vi "Publish.vi"(8 "error in (no error)":errorcluster, 10 "PublishRequest":refnum<class "PublishRequest.lvclass">, 11 "Mediator in":refnum<class "Mediator.lvclass">) -> (0 "error out":errorcluster, 3 "Mediator out":refnum<class "Mediator.lvclass">)   [LabVIEW 2019, in "Mediator.lvlib" / "Mediator.lvclass"]
doc: "<License>\nCopyright © 2017 Composed Systems, LLC | All rights reserved\nwww.composed.io\n\nAuthor: Ethan Stern <ethan.stern@composed.io>\n\nThis software is provided \"AS IS\" WITHOUT WARRANTIES, either express or implied, AND IS FOR EDUCATIONAL PURPOSES ONLY.\n</License>"
uses:
  <vilib>/gpm_packages/@cs/mva-core/Source/Mediator/Mediator/Mediator.lvclass
  <vilib>/gpm_packages/@cs/mva-core/Source/IMediator/PublishRequest/PublishRequest.lvclass
  <vilib>/gpm_packages/@cs/mva-core/Source/Mediator/Mediator/Mediator.lvclass/Mediator.ctl
  <vilib>/gpm_packages/@cs/mva-core/Source/IMediator/PublishRequest/PublishRequest.lvclass/PublishRequest.ctl
  <vilib>/gpm_packages/@cs/mva-core/Source/Mediator/TopicLookupTable/TopicLookupTable.lvclass/TopicLookupTable.ctl
  <vilib>/gpm_packages/@cs/mva-core/Source/Mediator/Topic Messages/Notify Subscribers Msg/Notify Subscribers Msg.lvclass/Notify Subscribers Msg.ctl
  <vilib>/ActorFramework/Message Enqueuer/Message Enqueuer.lvclass/Message Enqueuer.ctl
  <vilib>/ActorFramework/Message Enqueuer/Enqueue.vi
  <vilib>/gpm_packages/@cs/mva-core/Source/Mediator/Topic Messages/Notify Subscribers Msg/Notify Subscribers Msg.lvclass
  C:/Program Files/National Instruments/LabVIEW 2019/vi.lib/ActorFramework/Message/Message.lvclass
  <vilib>/gpm_packages/@cs/variant/Source/Format Type String.vi
  <vilib>/ActorFramework/Message Priority Queue/Priority Enqueue.vi
  <vilib>/ActorFramework/Message Enqueuer/Message Enqueuer.lvclass
  <vilib>/gpm_packages/@cs/mva-core/Source/Mediator/TopicLookupTable/TopicLookupTable.lvclass
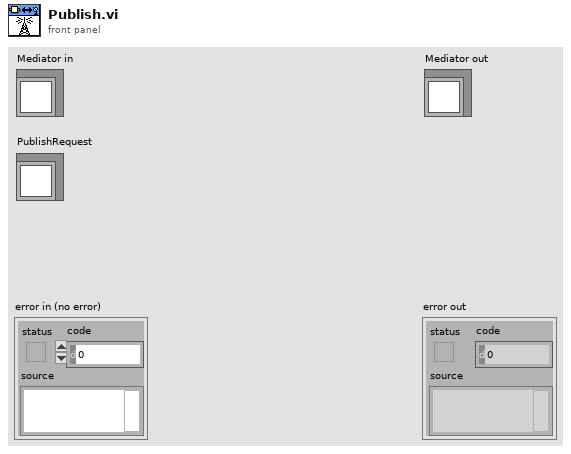
[diagram p1: front panel]
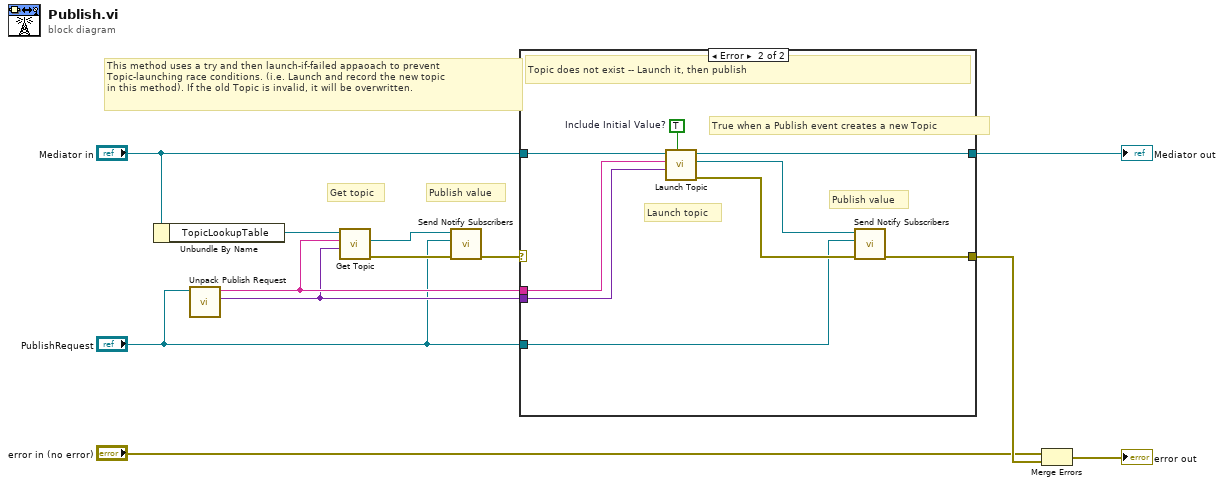
[diagram p0: block diagram]
diagram:
  # "Get topic"
  # "This method uses a try and then launch-if-failed appaoach to prevent\nTopic-launching race conditions. (i.e. Launch and record the new topic\nin this method). If the old Topic is invalid, it will be overwritten."
  # "Publish value"
  n1 = Unbundle By Name("Mediator in") -> ("TopicLookupTable"=w2:refnum<data-value>)
  n2 = call <vilib>:"Unpack Publish Request.vi"("PublishRequest In"="PublishRequest") -> ("Value"=w4:variant, "Datum Name"=w5:string)  [unwired: 7 in, 2 out]
  n3 = call <vilib>:"Get Topic.vi"("Topic Type"=w4, "Topic Name"=w5, "TopicLookupTable"=w2) -> ("error out"=w9:errorcluster, "Topic Enqueuer"=w12:refnum<class "Message Enqueuer.lvclass">)  [unwired: 6 in, 1 out]
  n4 = call <vilib>:"Send Notify Subscribers.vi"("error in (no error)"=w9, "PublishRequest"="PublishRequest", "Message Enqueuer"=w12) -> ("error out"=w11:errorcluster)  [unwired: 7 in, 1 out]
  n5 = case shown="Error" w11 {
    selector: w11 -> [w13 _]
    tunnel: "Mediator in" -> [w14 w23]
    tunnel: [w14 w21] -> w8
    tunnel: w5 -> [_ w19]
    tunnel: w4 -> [_ w18]
    tunnel: [w13 w22] -> w10
    tunnel: "PublishRequest" -> [_ w15]
    frame No Error {
      # "Topic exists -- Publish OK"
    }
    frame Error {
      w16 = TRUE  # Include Initial Value?
      # "True when a Publish event creates a new Topic"
      # "Launch topic"
      # "Publish value"
      # "Topic does not exist -- Launch it, then publish"
      n6 = call-dynamic "Launch Topic.vi"("Include Initial Value? (F)"=w16, "Type"=w18, "Datum Name"=w19, "Mediator in"=w23) -> ("error out"=w17:errorcluster, "New Topic Enqueuer"=w20:refnum<class "Message Enqueuer.lvclass">, "Mediator out"=w21:refnum<class "Mediator.lvclass">)  [unwired: 5 in]
      n7 = call <vilib>:"Send Notify Subscribers.vi"("error in (no error)"=w17, "PublishRequest"=w15, "Message Enqueuer"=w20) -> ("error out"=w22:errorcluster)  [unwired: 7 in, 1 out]
    }
  }
  "Mediator out" <- w8
  n8 = Merge Errors("error in (no error)", w10) -> (→"error out":errorcluster)
